vi "Driver Running on Server.vi"() -> (0 "Running on Server?":bool)   [LabVIEW 2011]
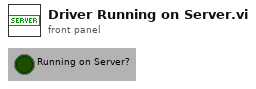
[diagram p1: front panel]
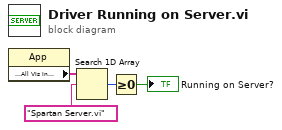
[diagram p0: block diagram]
diagram:
  n1 = property class="App"() -> ("Application:All VIs In Memory"=w1:string[])  [unwired: 2 in, 2 out]
  n2 = Search 1D Array(1D array=w1, element="Spartan Server.vi" ("y")) -> (index of element=w3:i32)  [unwired: 1 out]
  n3 = Greater Or Equal To 0?(x=w3) -> (x >= 0?=→"Running on Server?":bool)
